vi "Begin.vi"(8 "error in":errorcluster) -> (0 "error out":errorcluster)   [LabVIEW 2023]
doc: "Called before other user functions, this VI is expected to open initial I/O refnums, load in file data, and do all program initialization. Notice that the <B>error out</B> terminal is simply used for data flow. Wiring it to other structures or subVIs ensures that this VI runs first."
uses:
  <vilib>/Rock Robotics/WPI/DriverStation/WPI_DriverStationRobotMode2.ctl
  ctrl defs/ctrl pivot select.ctl
  ctrl defs/ctrl LIMELIGHT STREAM selector.ctl
  ctrl defs/ctrl LIMELIGHT LEDMODE selector.ctl
  ctrl defs/ctrl LIMELIGHT CAMMODE selector.ctl
  Robot Global Data.vi
  Global INIT.vi
  <vilib>/Rock Robotics/Network Tables/NT Write String Array.vi
  <vilib>/Rock Robotics/Network Tables/NT Write Boolean.vi
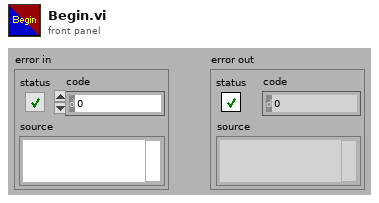
[diagram p1: front panel]
types:
  T1 = typedef "WPI_DriverStationRobotMode2.ctl" = enum16{"Autonomous Disabled", "Autonomous Enabled", "Teleop Disabled", "Teleop Enabled", "Disconnected", "Finish", "Test Disabled", "Test Enabled", "Emergency Stopped"}
  T2 = typedef "ctrl pivot select.ctl" = enum16{"geometric center", "CG", "FL", "FR", "RR", "RL", "other"}
  T3 = typedef "ctrl LIMELIGHT initialize.ctl" = cluster{"Installed?":bool, "pose":cluster{"X":dbl, "Y":dbl, "Z":dbl, "angle to horizon":dbl, "tx angle offset":dbl}}
  T4 = typedef "ctrl LIMELIGHT CAMMODE selector.ctl" = u16
  T5 = typedef "ctrl LIMELIGHT LEDMODE selector.ctl" = u16
  T6 = typedef "ctrl LIMELIGHT STREAM selector.ctl" = u16
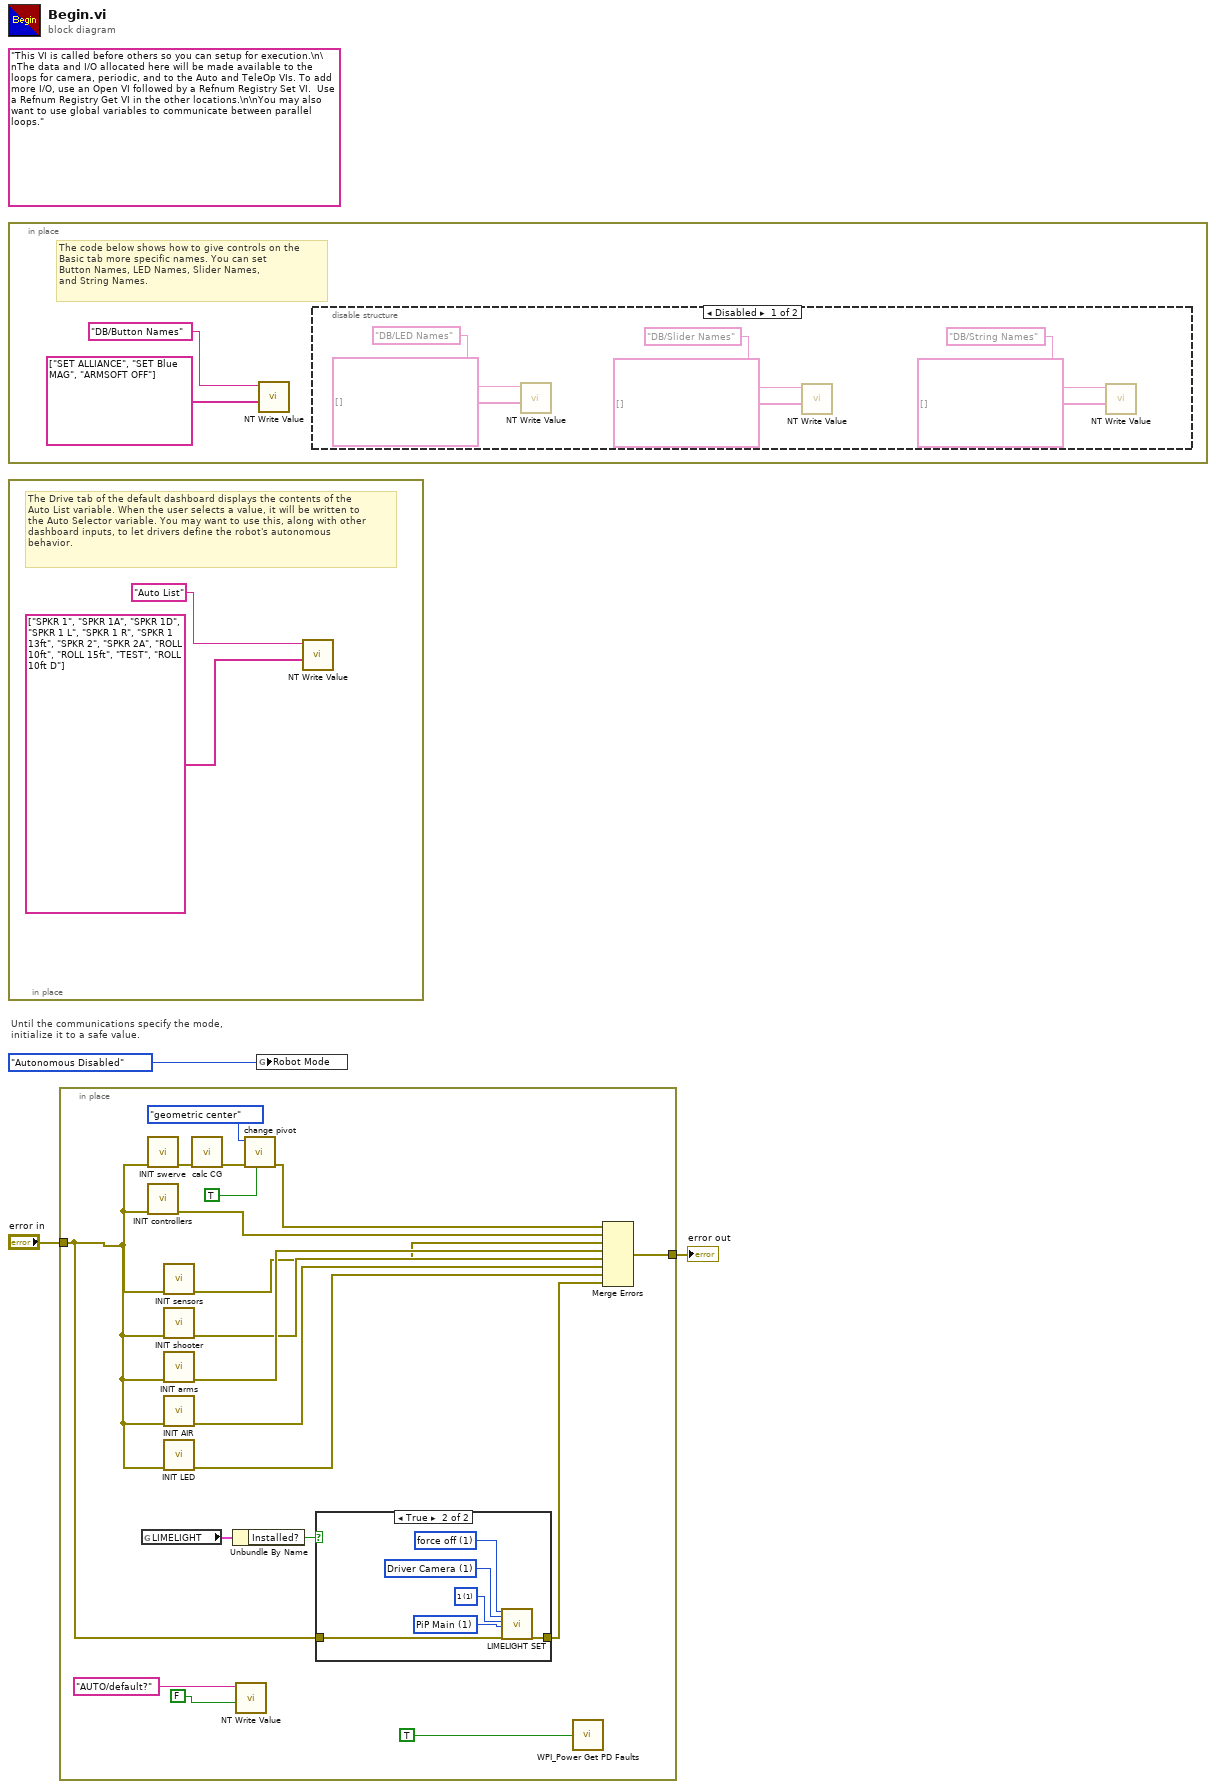
[diagram p0: block diagram]
diagram:
  (unwired) "This VI is called before others so you can setup for execution.\n\nThe data and I/O allocated here will be made available to the loops for camera, periodic, and to the Auto and TeleOp VIs. To add more I/O, use an Open VI followed by a Refnum Registry Set VI.  Use a Refnum Registry Get VI in the other locations.\n\nYou may also want to use global variables to communicate between parallel loops."
  # "Until the communications specify the mode,\ninitialize it to a safe value."
  n1 = in-place {
    # "The code below shows how to give controls on the\nBasic tab more specific names. You can set\nButton Names, LED Names, Slider Names,\nand String Names."
    n2 = call-poly <vilib>:"NT Write Value.vi"("value"=string[] ["SET ALLIANCE", "SET Blue MAG", "ARMSOFT OFF"], "name"="DB/Button Names" ("Name")) -> ()  [unwired: 9 in, 1 out]
    n3 = disable-structure shown="Disabled" {
      frame Disabled {
        n4 = call-poly <vilib>:"NT Write Value.vi"("value"=string[] [], "name"="DB/LED Names" ("Name")) -> ()  [unwired: 9 in, 1 out]
        n5 = call-poly <vilib>:"NT Write Value.vi"("value"=string[] [], "name"="DB/Slider Names" ("Name")) -> ()  [unwired: 9 in, 1 out]
        n6 = call-poly <vilib>:"NT Write Value.vi"("value"=string[] [], "name"="DB/String Names" ("Name")) -> ()  [unwired: 9 in, 1 out]
      }
      frame Enabled {
      }
    }
  }
  n7 = in-place {
    # "The Drive tab of the default dashboard displays the contents of the\nAuto List variable. When the user selects a value, it will be written to\nthe Auto Selector variable. You may want to use this, along with other\ndashboard inputs, to let drivers define the robot's autonomous\nbehavior."
    n8 = call-poly <vilib>:"NT Write Value.vi"("value"=string[] ["SPKR 1", "SPKR 1A", "SPKR 1D", "SPKR 1 L", "SPKR 1 R", "SPKR 1 13ft", "SPKR 2", "SPKR 2A", "ROLL 10ft", "ROLL 15ft", "TEST", "ROLL 10ft D"] ("String Array"), "name"="Auto List" ("Name")) -> ()  [unwired: 9 in, 1 out]
  }
  n9 = in-place {
    in-place-border: "error in" -> [w19]
    in-place-border: [w27] -> w1
    n10 = global read "Global INIT.vi" "LIMELIGHT"() -> (w17:T3)
    n11 = call "INIT swerve.vi"("error in (no error)"=w19) -> ("error out"=w32:errorcluster)  [unwired: 10 in]
    n12 = call "INIT controllers.vi"("error in (no error)"=w19) -> ("error out"=w28:errorcluster)  [unwired: 10 in]
    n13 = call "INIT sensors.vi"("error in (no error)"=w19) -> ("error out"=w22:errorcluster)  [unwired: 10 in]
    n14 = call "INIT shooter.vi"("error in (no error)"=w19) -> ("error out"=w23:errorcluster)  [unwired: 10 in]
    n15 = call "INIT arms.vi"("error in (no error)"=w19) -> ("error out"=w25:errorcluster)  [unwired: 10 in]
    n16 = call "INIT AIR.vi"("error in (no error)"=w19) -> ("error out"=w24:errorcluster)  [unwired: 10 in]
    n17 = call "INIT LED.vi"("error in (no error)"=w19) -> ("error out"=w26:errorcluster)  [unwired: 10 in]
    n18 = call "calc CG.vi"("error in (no error)"=w32) -> ("error out"=w31:errorcluster)  [unwired: 10 in]
    n19 = Unbundle By Name(w17) -> ("Installed?"=w16:bool)
    n20 = call-poly <vilib>:"NT Write Value.vi"("value"=FALSE, "name"="AUTO/default?") -> ()  [unwired: 9 in, 1 out]
    n21 = call "change pivot.vi"("force recalc?"=TRUE, "error in (no error)"=w31, "select pivot point"=ctrl_pivot_select."geometric center") -> ("error out"=w29:errorcluster)  [unwired: 8 in]
    n22 = case shown="True" w16 {
      tunnel: [w33 w39] -> w20
      tunnel: w19 -> [w33 w38]
      frame False {
      }
      frame True {
        w34 = T4 1 items=["Vision processor", "Driver Camera"] ("camMode")
        w35 = T5 1 items=["default to current pipeline", "force off", "force blink", "force on"] ("ledMode")
        w36 = T6 1 items=["standard side-by-side", "PiP Main", "PiP Secondary"] ("stream")
        w37 = u16 1 items=["0", "1", "2", "3", "4", "5", "6", "7", "8", "9"] ("pipeline")
        n23 = call "LIMELIGHT SET.vi"("ledMode"=w35, "camMode"=w34, "pipeline"=w37, "stream"=w36, "error in (no error)"=w38) -> ("error out"=w39:errorcluster)  [unwired: 14 in]
      }
    }
    n24 = call <vilib>:"WPI_Power Get PD Faults.vi"("Clear Sticky Faults"=TRUE) -> ()  [unwired: 11 in, 4 out]
    n25 = Merge Errors(w29, w28, w22, w25, w23, w24, w26, w20) -> (w27:errorcluster)
  }
  "error out" <- w1
  n26 = global write "Robot Global Data.vi" "Robot Mode"(WPI_DriverStationRobotMode2."Autonomous Disabled" ("Robot Mode")) -> ()
